vi "FTW-JSON-Object-SetElement-String.vi"(0 "JSON":refnum<class "FTW-Container.lvclass">, 5 "Key":string, 7 "Value":string, 11 "error in":errorcluster) -> (4 "JSON out":refnum<class "FTW-Container.lvclass">, 15 "error out":errorcluster)   [LabVIEW 2015]
uses:
  container/FTW-Container.lvclass
panel:
  # "Inputs"
  # "Outputs"
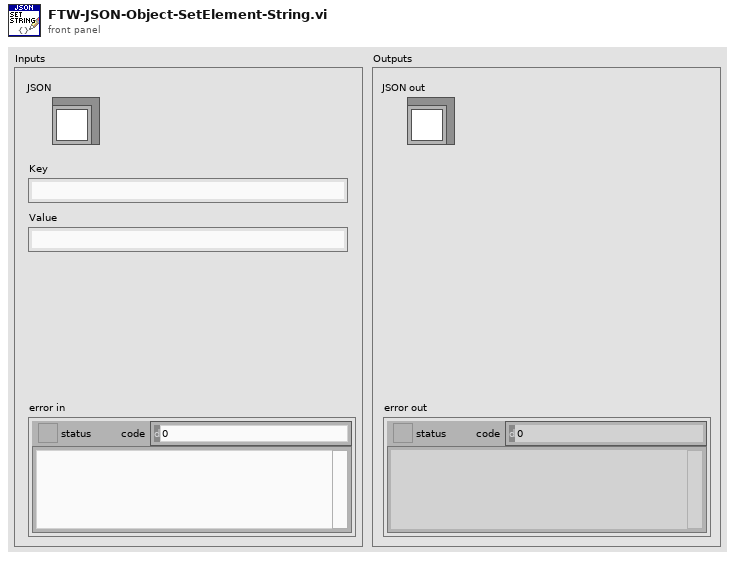
[diagram p1: front panel]
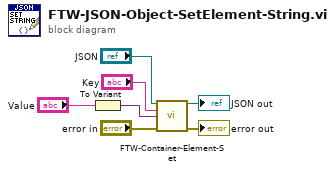
[diagram p0: block diagram]
diagram:
  n1 = To Variant(anything="Value") -> (Variant=w1:variant)
  n2 = call "FTW-Container-Element-Set.vi"("FTW-Container In"="JSON", "Element Name"="Key", "Value"=w1, "error in"="error in") -> ("FTW-Container Out"=→"JSON out":refnum<class "FTW-Container.lvclass">, "error out"=→"error out":errorcluster)  [unwired: 9 in, 1 out]
